vi "DeCoF terminal screen emulator.vi"(4 "time stamp":bool, 5 "history in":string, 6 "remember cursor in":i32, 7 "new string":string) -> (1 "history out":string, 2 "remember cursor out":i32)   [LabVIEW 2013]
doc: "This VI emulates a (VT100) terminal by appending characters to the string \"history in\" at the position given by \"remeber cursor in\". The \"new string\" is supposed to be received from the laser. It usally contains regular characters like letters and numerical digits but also some special characters and character sequences like backspace, new line, cursor left, cursor right, etc. or toggling between insert and overwrite mode. These are coded in VT100 style. The modified string and the new cursor position are returned in \"history out\" and \"remember cursor out\", respectively."
uses:
  subVIs/DeCoF VT100 parser state.ctl
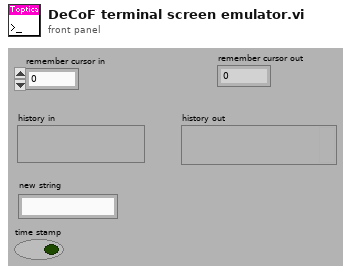
[diagram p1: front panel]
types:
  T1 = typedef "DeCoF VT100 parser state.ctl" = enum16{"ESC received", "[ received", "parameter received", "regular input"}
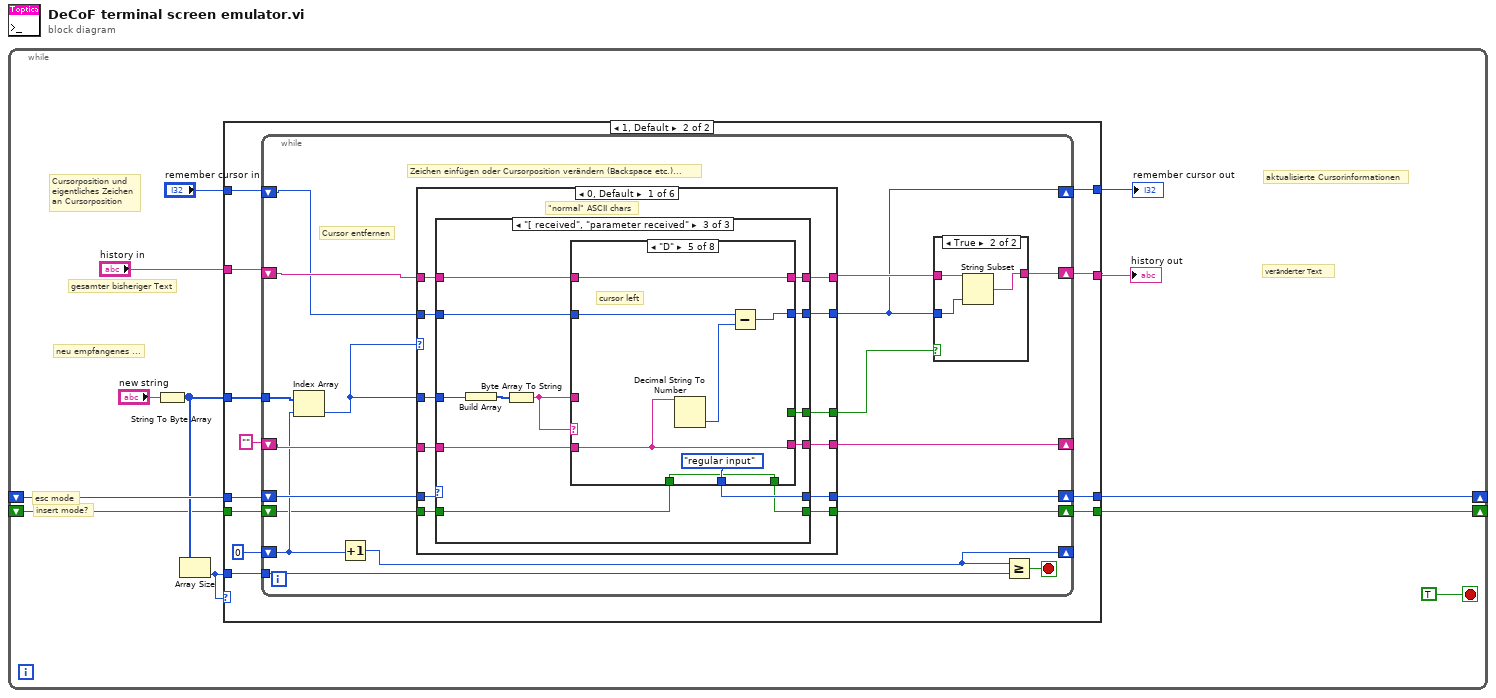
[diagram p0: block diagram]
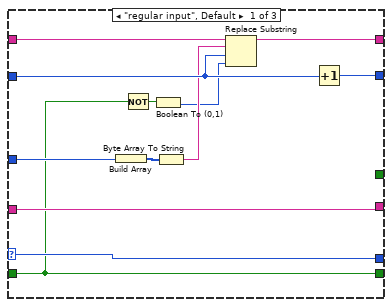
[diagram p4: hidden frame]
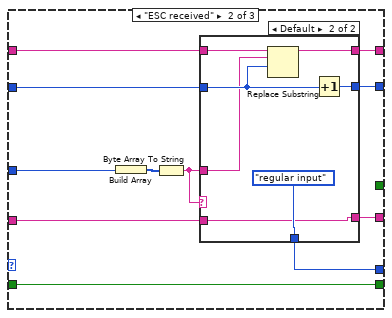
[diagram p5: hidden frame]
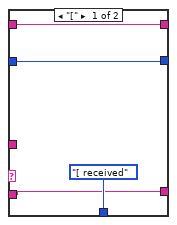
[diagram p6: hidden frame]
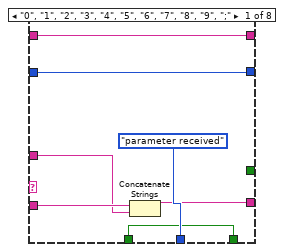
[diagram p7: hidden frame]
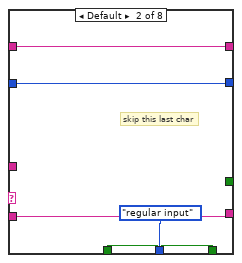
[diagram p8: hidden frame]
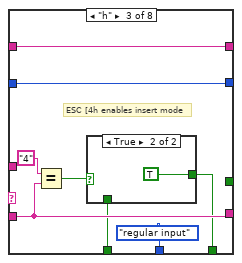
[diagram p9: hidden frame]
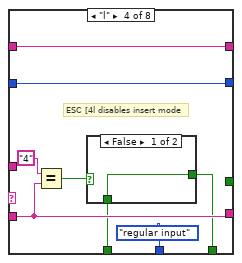
[diagram p11: hidden frame]
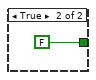
[diagram p12: hidden frame]
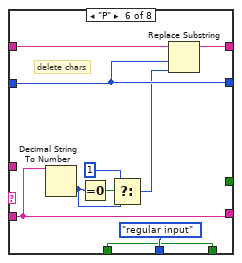
[diagram p13: hidden frame]
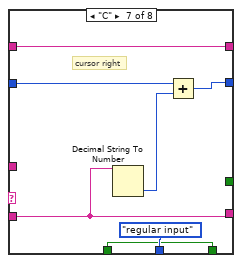
[diagram p14: hidden frame]
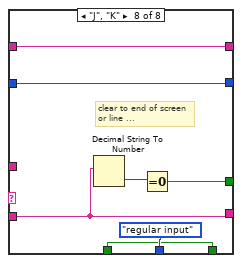
[diagram p15: hidden frame]
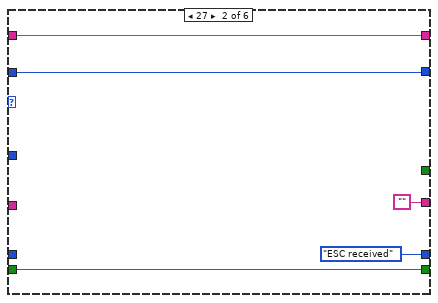
[diagram p16: hidden frame]
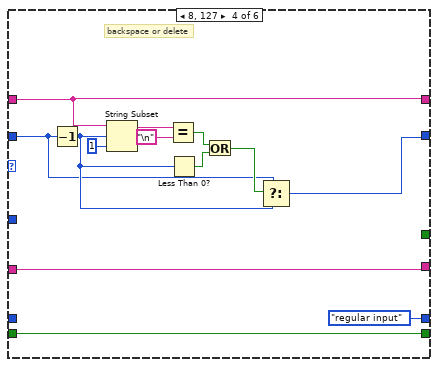
[diagram p18: hidden frame]
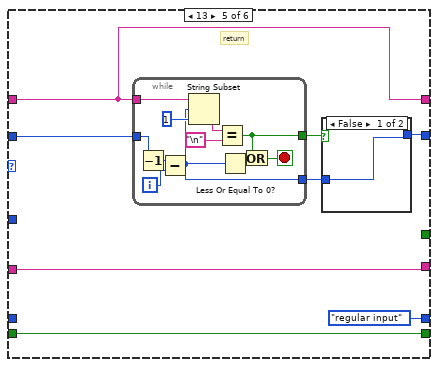
[diagram p19: hidden frame]
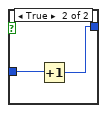
[diagram p20: hidden frame]
diagram:
  n1 = while {
    shift-right: [w5] -> _
    shift-left: _ -> [w6]
    shift-right: [w2] -> _
    shift-left: _ -> [w1]
    stop <- TRUE stop-if-true
    # "esc mode"
    # "insert mode?"
    # "veränderter Text"
    # "aktualisierte Cursorinformationen"
    # "neu empfangenes ..."
    # "gesamter bisheriger Text"
    # "Cursorposition und\neigentliches Zeichen\nan Cursorposition"
    n2 = String To Byte Array(string="new string") -> (unsigned byte array=w4:u8[])
    n3 = Array Size(array=w4) -> (size(s)=w3:i32)
    n4 = case shown="1, Default" w3 {
      tunnel: "remember cursor in" -> [w16 w28]
      tunnel: "history in" -> [w15 w27]
      tunnel: [w16 w26] -> w9
      tunnel: [w15 w25] -> w8
      tunnel: w6 -> [w14 w24]
      tunnel: [w14 w23] -> w5
      tunnel: w4 -> [_ w20]
      tunnel: w3 -> [_ w19]
      tunnel: [w13 w18] -> w2
      tunnel: w1 -> [w13 w17]
      frame 0 {
      }
      frame 1, Default {
        n5 = while {
          tunnel: w20 -> [w35]
          shift-right: [w31] -> w26
          shift-left: w28 -> [w32]
          shift-right: [w42] -> w25
          shift-left: w27 -> [w40]
          shift-right: [w46] -> w23
          shift-left: w24 -> [w45]
          shift-right: [w43] -> _
          shift-left: "" -> [w44]
          shift-right: [w37] -> _
          shift-left: 0 -> [w34]
          tunnel: w19 -> [w39]
          shift-right: [w30] -> w18
          shift-left: w17 -> [w29]
          stop <- w38 stop-if-true
          # "Zeichen einfügen oder Cursorposition verändern (Backspace etc.)..."
          # "Cursor entfernen"
          n6 = Index Array(array=w35, index=w34) -> (element=w33:u8)
          n7 = Increment(x=w34) -> (x+1=w37:i32)
          n8 = case shown="0, Default" w33 {
            tunnel: w40 -> [w61 w177 w182 w185 w200 w226]
            tunnel: [w62 w177 w182 w185 w200 w222] -> w36
            tunnel: w32 -> [w60 w176 w181 w184 w197 _]
            tunnel: [w59 w176 w181 w187 w201 w224] -> w31
            tunnel: w33 -> [w58 _ _ _ _ _]
            tunnel: [w56 DeCoF_VT100_parser_state."ESC received" ("Enum") w179 DeCoF_VT100_parser_state."regular input" ("Enum") DeCoF_VT100_parser_state."regular input" ("Enum") DeCoF_VT100_parser_state."regular input" ("Enum")] -> w46
            tunnel: w45 -> [w57 _ w179 _ _ _]
            tunnel: w44 -> [w55 _ w180 w188 w198 w219]
            tunnel: [w54 "" w180 w188 w198 w219] -> w43
            tunnel: [w53 _ _ _ _ _] -> w41
            tunnel: [w52 w173 w178 w183 w196 w218] -> w30
            tunnel: w29 -> [w51 w173 w178 w183 w196 w218]
            frame 0, Default {
              # "\"normal\" ASCII chars"
              n9 = case shown="\"[ received\", \"parameter received\"" w57 {
                selector: w57 -> [w68 _ _]
                tunnel: [w74 w85 w109] -> w62
                tunnel: w61 -> [w73 w84 w108]
                tunnel: w60 -> [w72 w83 w107]
                tunnel: [w71 w82 w106] -> w59
                tunnel: w58 -> [w66 w80 w104]
                tunnel: [w68 w78 w102] -> w56
                tunnel: w55 -> [w67 w77 w101]
                tunnel: [w67 w76 w100] -> w54
                tunnel: [_ _ w99] -> w53
                tunnel: [w65 w75 w98] -> w52
                tunnel: w51 -> [w65 w75 w97]
                frame "regular input", Default {
                  n10 = Build Array(w66) -> (w70:u8[])
                  n11 = Not(x=w65) -> (.not. x?=w64:bool)
                  n12 = Boolean To (0,1)(Boolean=w64) -> (0, 1=w63:i16)
                  n13 = Byte Array To String(unsigned byte array=w70) -> (string=w69:string)
                  n14 = Replace Substring(2:w63, 3:w72, 4:w69, 5:w73) -> (1:w74:string)  [unwired: 1 out]
                  n15 = Increment(x=w72) -> (x+1=w71:i32)
                }
                frame "ESC received" {
                  n16 = Build Array(w80) -> (w81:u8[])
                  n17 = Byte Array To String(unsigned byte array=w81) -> (string=w79:string)
                  n18 = case shown="Default" w79 {
                    tunnel: [w89 w96] -> w85
                    tunnel: w84 -> [w89 w95]
                    tunnel: w83 -> [w88 w94]
                    tunnel: [w88 w93] -> w82
                    tunnel: w79 -> [_ w92]
                    tunnel: [DeCoF_VT100_parser_state."[ received" ("Enum") DeCoF_VT100_parser_state."regular input" ("Enum")] -> w78
                    tunnel: w77 -> [w86 w90]
                    tunnel: [w86 w90] -> w76
                    frame "[" {
                    }
                    frame Default {
                      n19 = Replace Substring(3:w94, 4:w92, 5:w95) -> (1:w96:string)  [unwired: 1 in, 1 out]
                      n20 = Increment(x=w94) -> (x+1=w93:i32)
                    }
                  }
                }
                frame "[ received", "parameter received" {
                  n21 = Build Array(w104) -> (w105:u8[])
                  n22 = Byte Array To String(unsigned byte array=w105) -> (string=w103:string)
                  n23 = case shown="\"D\"" w103 {
                    tunnel: [w116 w119 w127 w137 w144 w154 w161 w171] -> w109
                    tunnel: w108 -> [w116 w119 w127 w137 w144 w155 w161 w171]
                    tunnel: w107 -> [w115 w120 w128 w138 w147 w153 w164 w169]
                    tunnel: [w115 w120 w128 w138 w145 w153 w162 w169] -> w106
                    tunnel: w103 -> [w112 _ _ _ _ _ _ _]
                    tunnel: [DeCoF_VT100_parser_state."parameter received" ("Enum") DeCoF_VT100_parser_state."regular input" ("Enum") DeCoF_VT100_parser_state."regular input" ("Enum") DeCoF_VT100_parser_state."regular input" ("Enum") DeCoF_VT100_parser_state."regular input" ("Enum") DeCoF_VT100_parser_state."regular input" ("Enum") DeCoF_VT100_parser_state."regular input" ("Enum") DeCoF_VT100_parser_state."regular input" ("Enum")] -> w102
                    tunnel: w101 -> [w113 w118 w126 w136 w143 w157 w160 w170]
                    tunnel: [w111 w118 w126 w136 w143 w157 w160 w170] -> w100
                    tunnel: [_ _ _ _ _ _ _ w167] -> w99
                    tunnel: [w110 w117 w123 w133 w142 w156 w159 w166] -> w98
                    tunnel: w97 -> [w110 w117 w122 w132 w142 w156 w159 w166]
                    frame "0", "1", "2", "3", "4", "5", "6", "7", "8", "9", ";" {
                      n24 = Concatenate Strings(w113, w112) -> (w111:string)
                    }
                    frame Default {
                      # "skip this last char"
                    }
                    frame "h" {
                      # "ESC [4h enables insert mode"
                      n25 = Equal?(x="4", y=w126) -> (x = y?=w124:bool)
                      n26 = case shown="True" w124 {
                        tunnel: [w130 TRUE] -> w123
                        tunnel: w122 -> [w130 _]
                        frame False {
                        }
                        frame True {
                        }
                      }
                    }
                    frame "l" {
                      # "ESC [4l disables insert mode"
                      n27 = Equal?(x="4", y=w136) -> (x = y?=w134:bool)
                      n28 = case shown="False" w134 {
                        tunnel: [w140 FALSE] -> w133
                        tunnel: w132 -> [w140 _]
                        frame False {
                        }
                        frame True {
                        }
                      }
                    }
                    frame "D" {
                      # "cursor left"
                      n29 = Decimal String To Number(string=w143) -> (number=w146:i32)  [unwired: 2 in, 1 out]
                      n30 = Subtract(x=w147, y=w146) -> (x-y=w145:i32)
                    }
                    frame "P" {
                      # "delete chars"
                      n31 = Decimal String To Number(string=w157) -> (number=w150:i32)  [unwired: 2 in, 1 out]
                      n32 = Equal To 0?(x=w150) -> (x = 0?=w152:bool)
                      n33 = Select(t=1, s=w152, f=w150) -> (s? t:f=w151:i32)
                      n34 = Replace Substring(2:w151, 3:w153, 5:w155) -> (1:w154:string)  [unwired: 1 in, 1 out]
                    }
                    frame "C" {
                      # "cursor right"
                      n35 = Decimal String To Number(string=w160) -> (number=w163:i32)  [unwired: 2 in, 1 out]
                      n36 = Add(x=w164, y=w163) -> (x+y=w162:i32)
                    }
                    frame "J", "K" {
                      # "clear to end of screen\nor line ..."
                      n37 = Decimal String To Number(string=w170) -> (number=w168:i32)  [unwired: 2 in, 1 out]
                      n38 = Equal To 0?(x=w168) -> (x = 0?=w167:bool)
                    }
                  }
                }
              }
            }
            frame 27 {
            }
            frame 7 {
              # "BINGGGG !!"
            }
            frame 8, 127 {
              # "backspace or delete"
              n39 = Decrement(x=w184) -> (x-1=w190:i32)
              n40 = String Subset(string=w185, offset (0)=w190, length (rest)=1 ("length (rest)")) -> (substring=w194:string)
              n41 = Equal?(x=w194, y="\n") -> (x = y?=w191:bool)
              n42 = Less Than 0?(x=w190) -> (x < 0?=w192:bool)
              n43 = Or(x=w191, y=w192) -> (x .or. y?=w186:bool)
              n44 = Select(t=w184, s=w186, f=w190) -> (s? t:f=w187:i32)
            }
            frame 13 {
              # "return"
              n45 = while {
                tunnel: [w205] -> w203
                tunnel: [w206] -> w202
                tunnel: w200 -> [w214]
                tunnel: w197 -> [w204]
                i -> [w213]
                stop <- w208 stop-if-true
                n46 = Decrement(x=w204) -> (x-1=w207:i32)
                n47 = Subtract(x=w207, y=w213) -> (x-y=w206:i32)
                n48 = String Subset(string=w214, offset (0)=w206, length (rest)=1 ("length (rest)")) -> (substring=w211:string)
                n49 = Equal?(x=w211, y="\n") -> (x = y?=w205:bool)
                n50 = Less Or Equal To 0?(x=w206) -> (x <= 0?=w209:bool)
                n51 = Or(x=w205, y=w209) -> (x .or. y?=w208:bool)
              }
              n52 = case shown="False" w203 {
                tunnel: w202 -> [w215 w217]
                tunnel: [w215 w216] -> w201
                frame False {
                }
                frame True {
                  n53 = Increment(x=w217) -> (x+1=w216:i32)
                }
              }
            }
            frame 10 {
              # "new line"
              n54 = Concatenate Strings(w226, "\n" ("Substring")) -> (w223:string)
              n55 = case shown="False" "time stamp" {
                tunnel: w223 -> [w227 w236]
                tunnel: [w227 w235] -> w222
                frame False {
                }
                frame True {
                  n56 = Get Date/Time In Seconds() -> (seconds since 1Jan1904=w228:timestamp)
                  n57 = To Double Precision Float(number=w228) -> (double precision float=w230:dbl)
                  n58 = Get Date/Time String(seconds (now)=w230, want seconds? (F)=TRUE) -> (time string=w232:string)  [unwired: 1 in, 1 out]
                  n59 = Concatenate Strings(w236, "[" ("Substring"), w232, "]" ("Substring"), "\t") -> (w235:string)
                }
              }
              n60 = String Length(string=w222) -> (length=w224:i32)
            }
          }
          n61 = case shown="True" w41 {
            tunnel: w36 -> [w47 w50]
            tunnel: [w47 w49] -> w42
            tunnel: w31 -> [_ w48]
            frame False {
            }
            frame True {
              n62 = String Subset(string=w50, length (rest)=w48) -> (substring=w49:string)  [unwired: 1 in]
            }
          }
          n63 = Greater Or Equal?(x=w37, y=w39) -> (x >= y?=w38:bool)
        }
      }
    }
    "remember cursor out" <- w9
    "history out" <- w8
  }
